vi "GL_HomeSWLims.vi"(7 "SoftwareLims?":bool, 8 "error in":errorcluster, 10 "Axis IN":T1 items=["Axis 1", "Axis 2", "Axis 3", "Axis 4", "Axis 5", "Axis 6", "Axis 7", "Axis 8"], 11 "Galil.IGalil":refnum<k7>) -> (0 "error out":errorcluster, 2 "Axis Out":T1 items=["Axis 1", "Axis 2", "Axis 3", "Axis 4", "Axis 5", "Axis 6", "Axis 7", "Axis 8"], 3 "ref out":refnum<k7>)   [LabVIEW 2022 SP3]
uses:
  GL Axis Control.ctl
  Command Menu.ctl
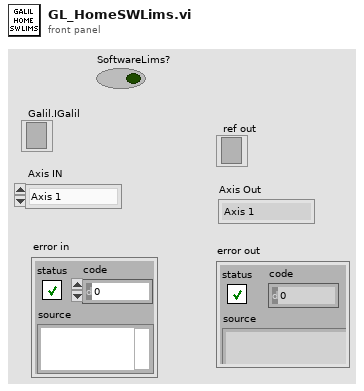
[diagram p1: front panel]
types:
  T1 = typedef "GL Axis Control.ctl" = u16
  T2 = typedef "Command Menu.ctl" = enum16{"CommandPassThrough", "Abort Motion", "Define Pos", "Velocity", "Acceleration", "Deceleration", "Position Rel", "Postion Abs", "Begin Move", "After Move", "Home", "KI", "KD", "KP", "IL", "Config I/O", "Set Bit", "Clear Bit", "Motor Off", "Moto On", "Status", "Execute", "Halt Execute", "HX Status", "Tell Velocity", "Check Motion", "BreakPoint", "Tell Position", "Current Code Line", "Tell Switches", "OC Force On", "OC Off", "Pos Soft Limit", "Rev Soft Limit"}
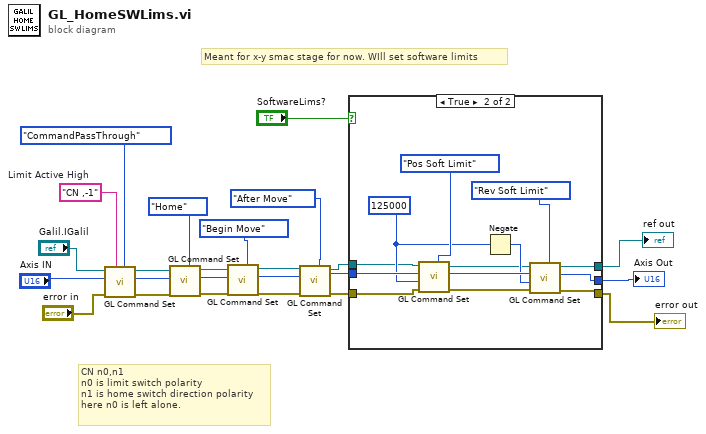
[diagram p0: block diagram]
diagram:
  w9 = "CN ,-1"  # Limit Active High
  # "Meant for x-y smac stage for now. WIll set software limits"
  # "CN n0,n1\nn0 is limit switch polarity\nn1 is home switch direction polarity\nhere n0 is left alone."
  n1 = call "GL Command Set.vi"("Command"=Command_Menu."CommandPassThrough", "Text Input"=w9, "error in (no error)"="error in", "Axis"="Axis IN", "Galil.IGalil"="Galil.IGalil") -> ("error out"=w11:errorcluster, "Axis Out"=w10:T1, "ref out"=w12:refnum<k7>)  [unwired: 2 in, 2 out]
  n2 = call "GL Command Set.vi"("Command"=Command_Menu."Home", "error in (no error)"=w11, "Axis"=w10, "Galil.IGalil"=w12) -> ("error out"=w21:errorcluster, "Axis Out"=w18:T1, "ref out"=w22:refnum<k7>)  [unwired: 3 in, 2 out]
  n3 = call "GL Command Set.vi"("Command"=Command_Menu."Begin Move", "error in (no error)"=w21, "Axis"=w18, "Galil.IGalil"=w22) -> ("error out"=w19:errorcluster, "Axis Out"=w17:T1, "ref out"=w20:refnum<k7>)  [unwired: 3 in, 2 out]
  n4 = call "GL Command Set.vi"("Command"=Command_Menu."After Move", "error in (no error)"=w19, "Axis"=w17, "Galil.IGalil"=w20) -> ("error out"=w13:errorcluster, "Axis Out"=w15:T1, "ref out"=w4:refnum<k7>)  [unwired: 3 in, 2 out]
  n5 = case shown="True" "SoftwareLims?" {
    tunnel: w15 -> [w25 w38]
    tunnel: w13 -> [w27 w34]
    tunnel: [w26 w30] -> w3
    tunnel: [w27 w29] -> w1
    tunnel: w4 -> [w26 w31]
    tunnel: [w25 w28] -> w2
    frame False {
    }
    frame True {
      w36 = 125000 ("Value")
      n6 = call "GL Command Set.vi"("Command"=Command_Menu."Pos Soft Limit", "error in (no error)"=w34, "Value"=w36, "Axis"=w38, "Galil.IGalil"=w31) -> ("error out"=w33:errorcluster, "Axis Out"=w37:T1, "ref out"=w32:refnum<k7>)  [unwired: 2 in, 2 out]
      n7 = Negate(x=w36) -> (-x=w35:i32)
      n8 = call "GL Command Set.vi"("Command"=Command_Menu."Rev Soft Limit", "error in (no error)"=w33, "Value"=w35, "Axis"=w37, "Galil.IGalil"=w32) -> ("error out"=w29:errorcluster, "Axis Out"=w28:T1, "ref out"=w30:refnum<k7>)  [unwired: 2 in, 2 out]
    }
  }
  "Axis Out" <- w2
  "error out" <- w1
  "ref out" <- w3
